vi "新剖面数据上传.vi"(11 "错误输入（无错误）":errorcluster) -> (15 "error out":errorcluster)   [LabVIEW 2016, in "数据传输系统-02.lvlib"]
uses:
  <vilib>/Utility/config.llb/Write Key (String).vi
  <vilib>/Utility/config.llb/Read Key (String).vi
  <vilib>/Utility/config.llb/NI_LVConfig.lvlib
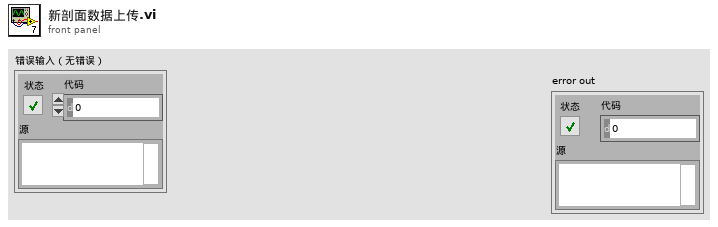
[diagram p1: front panel]
types:
  T1 = cluster{"setini":string, "sysini":string, "hechaini":string, "actualwrite":string, "actualread":string, "datasent":string, "反控命令信息队列":string, "反控与仪器交互":string}
  T2 = typedef "NI_LVConfig.lvlib/Config Data RefNum.ctl" = refnum<k1>
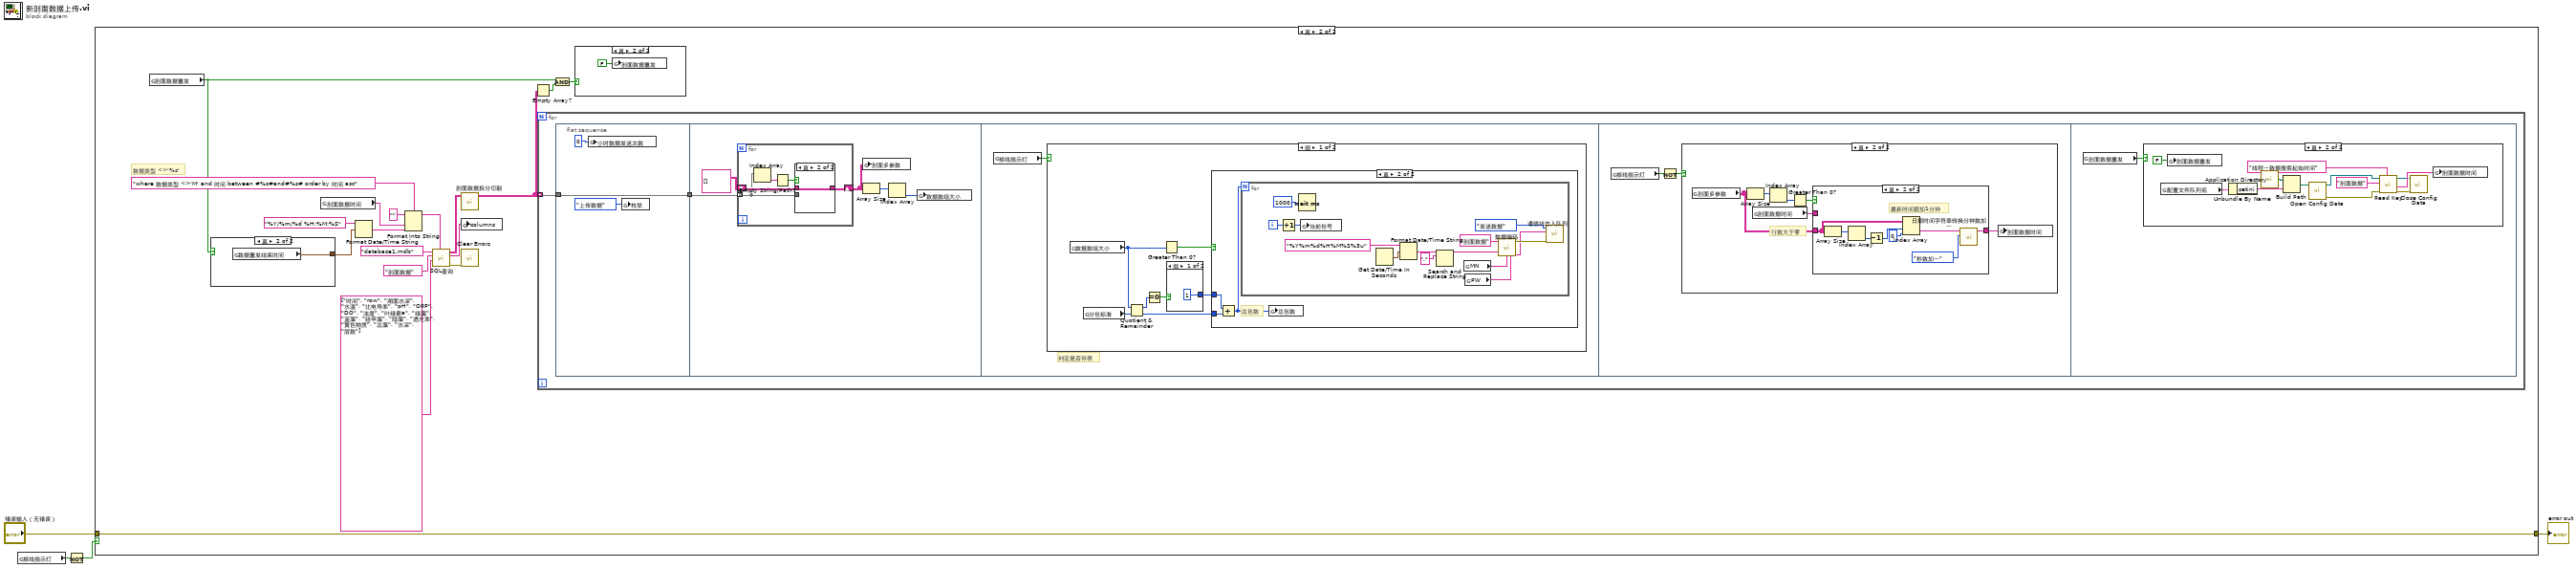
[diagram p0: block diagram]
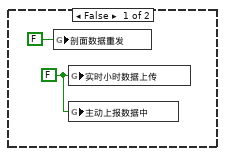
[diagram p2: hidden frame]
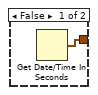
[diagram p4: hidden frame]
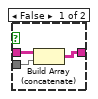
[diagram p5: hidden frame]
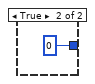
[diagram p6: hidden frame]
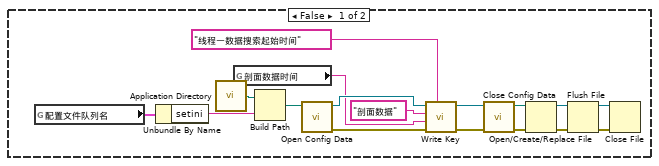
[diagram p11: hidden frame]
diagram:
  n1 = global read "全局 数据发送重叠.vi" "掉线指示灯"() -> (w4:bool)
  n2 = Not(x=w4) -> (.not. x?=w1:bool)
  n3 = case shown="真" w1 {
    tunnel: [_ w24] -> w3
    tunnel: "错误输入（无错误）" -> [_ w24]
    frame False {
      w6 = FALSE ("小时数据上传")
      n4 = global write "断电保存全局.vi" "剖面数据重发"(FALSE ("剖面数据重发")) -> ()
      n5 = global write "全局1.vi" "实时小时数据上传"(w6) -> ()
      n6 = global write "全局 数据发送重叠.vi" "主动上报数据中"(w6) -> ()
    }
    frame True {
      # "数据类型 <>'%s'"
      n7 = global read "断电保存全局.vi" "剖面数据重发"() -> (w7:bool)
      n8 = case shown="真" w7 {
        tunnel: [w26 w27] -> w11
        frame False {
          n9 = Get Date/Time In Seconds() -> (seconds since 1Jan1904=w26:timestamp)
        }
        frame True {
          n10 = global read "断电保存全局.vi" "数据重发结束时间"() -> (w27:timestamp)
        }
      }
      n11 = global read "全局 水样时间.vi" "剖面数据时间"() -> (w17:string)
      n12 = Format Date/Time String(time format string (%c)="%Y/%m/%d %H:%M:%S" ("时间格式字符串(%c)"), seconds (now)=w11) -> (date/time string=w16:string)  [unwired: 1 in]
      n13 = Format Into String(format string="where 数据类型 <>'M' and 时间 between #%s#and#%s# order by 时间 asc" ("condition"), initial string="" ("初始字符串"), w17, w16) -> (resulting string=w15:string)  [unwired: 1 in, 1 out]
      n14 = call "SQL查询.vi"("condition"=w15, "columns"=string[] ["时间", "row", "湖面水深", "水温", "比电导率", "pH", "ORP", "DO", "浊度", "叶绿素a", "绿藻", "蓝藻", "硅甲藻", "隐藻", "透光率", "黄色物质", "总藻", "水深", "层数"], "table输入"="剖面数据", "database"="database1.mdb") -> ("error out"=w13:errorcluster, "columns输出"=w14:string[], "data"=w23:string[][])  [unwired: 4 in, 1 out]
      n15 = call "剖面数据拆分切割.vi"("剖面多参数输入"=w23) -> ("剖面多参数输出"=w10:string[][][])  [unwired: 10 in]
      n16 = global write "全局 所有参数.vi" "columns"(w14) -> ()
      n17 = call <vilib>:"Clear Errors.vi"("error in (no error)"=w13) -> ()  [unwired: 5 in, 2 out]
      n18 = Empty Array?(array=w10) -> (empty?=w9:bool)
      n19 = for {
        tunnel: w10 -> [w29] mode=indexing
        n20 = flat-sequence {
          tunnel: w29 -> [w32]
          tunnel: [w32] -> w28
          tunnel: w28 -> [w35]
          frame #0 {
            n21 = global write "全局 小时数据发送次数.vi" "小时数据发送次数"(0 ("小时数据发送次数")) -> ()
            n22 = global write "全局1.vi" "枚举"(enum16{"返回请求应答", "上传数据", "返回执行结果"}."上传数据" ("枚举")) -> ()
          }
          frame #1 {
            n23 = for {
              tunnel: w35 -> [w40] mode=indexing
              shift-right: [w41] -> w33
              shift-left: string[][] [] ("剖面多参数输入") -> [w42]
              n24 = Index Array(array=w40) -> (element=w39:string)  [unwired: 1 in]
              n25 = Empty String/Path?(string/path=w39) -> (empty?=w38:bool)
              n26 = case shown="真" w38 {
                tunnel: w42 -> [w45 w46]
                tunnel: w40 -> [w44 _]
                tunnel: [w43 w46] -> w41
                frame False {
                  n27 = Build Array (concatenate)(w45, w44) -> (w43:string[][])
                }
                frame True {
                }
              }
            }
            n28 = global write "全局 所有参数.vi" "剖面多参数"(w33) -> ()
            n29 = Array Size(array=w33) -> (size(s)=w36:i32[])
            n30 = Index Array(array=w36) -> (element=w37:i32)  [unwired: 1 in]
            n31 = global write "全局 数据数组大小.vi" "数据数组大小"(w37) -> ()
          }
          frame #2 {
            # "判定是否存表"
            n32 = global read "全局 数据发送重叠.vi" "掉线指示灯"() -> (w47:bool)
            n33 = case shown="假" w47 {
              frame False {
                n34 = global read "全局 数据数组大小.vi" "数据数组大小"() -> (w53:i32)
                n35 = global read "全局 数据数组大小.vi" "分包标准"() -> (w51:i32)
                n36 = Quotient & Remainder(x=w53, y=w51) -> (x-y*floor(x/y)=w50:i32, floor(x/y)=w52:i32)
                n37 = Equal To 0?(x=w50) -> (x = 0?=w49:bool)
                n38 = Greater Than 0?(x=w53) -> (x > 0?=w54:bool)
                n39 = case shown="假" w49 {
                  tunnel: [1 ("x") 0 ("x")] -> w48
                  frame False {
                  }
                  frame True {
                  }
                }
                n40 = case shown="真" w54 {
                  tunnel: w52 -> [_ w59]
                  tunnel: w48 -> [_ w57]
                  frame False {
                  }
                  frame True {
                    # "总包数"
                    n41 = Add(x=w57, y=w59) -> (x+y=w58:i32)
                    n42 = for {
                      N: w58 -> [_]
                      i -> [w63]
                      n43 = Increment(x=w63) -> (x+1=w62:i32)
                      n44 = Wait (ms)(milliseconds to wait=u32 1000 ("等待时间（毫秒）")) -> ()  [unwired: 1 out]
                      n45 = global write "全局 数据数组大小.vi" "当前包号"(w62) -> ()
                      n46 = Get Date/Time In Seconds() -> (seconds since 1Jan1904=w71:timestamp)
                      n47 = Format Date/Time String(time format string (%c)="%Y%m%d%H%M%S%3u" ("时间格式字符串(%c)"), seconds (now)=w71) -> (date/time string=w70:string)  [unwired: 1 in]
                      n48 = Search and Replace String(input string=w70, search string="." ("搜索字符串")) -> (result string=w68:string)  [unwired: 6 in, 3 out]
                      n49 = global read "断电保存全局.vi" "MN"() -> (w67:string)
                      n50 = global read "断电保存全局.vi" "PW"() -> (w66:string)
                      n51 = call "数据编码.vi"("table输入"="剖面数据" ("新元素/子数组"), "QN"=w68, "MN"=w67, "PW"=w66) -> ("错误常量"=w65:errorcluster, "通讯包字符串"=w60:string)  [unwired: 10 in]
                      n52 = call "通信状态入队列.vi"("错误输入（无错误）"=w65, "发送报文"=w60, "枚举"=enum16{"打开连接", "发送数据", "读取数据", "数据处理", "关闭连接"}."发送数据") -> ()  [unwired: 8 in, 1 out]
                    }
                    n53 = global write "全局 数据数组大小.vi" "总包数"(w58) -> ()
                  }
                }
              }
              frame True {
              }
            }
          }
          frame #3 {
            n54 = global read "全局 数据发送重叠.vi" "掉线指示灯"() -> (w74:bool)
            n55 = Not(x=w74) -> (.not. x?=w75:bool)
            n56 = case shown="真" w75 {
              frame False {
              }
              frame True {
                # "行数大于零"
                n57 = global read "全局 所有参数.vi" "剖面多参数"() -> (w80:string[][])
                n58 = Array Size(array=w80) -> (size(s)=w77:i32[])
                n59 = global read "全局 水样时间.vi" "剖面数据时间"() -> (w81:string)
                n60 = Index Array(array=w77) -> (element=w78:i32)  [unwired: 1 in]
                n61 = Greater Than 0?(x=w78) -> (x > 0?=w79:bool)
                n62 = case shown="真" w79 {
                  tunnel: w80 -> [_ w87]
                  tunnel: [w82 w84] -> w76
                  tunnel: w81 -> [w82 _]
                  frame False {
                  }
                  frame True {
                    # "最新时间戳加1分钟"
                    n63 = Array Size(array=w87) -> (size(s)=w89:i32[])
                    n64 = Index Array(array=w89) -> (element=w88:i32)  [unwired: 1 in]
                    n65 = Decrement(x=w88) -> (x-1=w86:i32)
                    n66 = Index Array(array=w87, index (row)=w86, index (col)=0 ("禁用的索引 (列)")) -> (element=w90:string)
                    n67 = call "日期时间字符串转换分钟数加一.vi"("枚举"=enum16{"分钟数加一", "秒数加一", "小时数加一"}."秒数加一", "data[0]"=w90) -> ("日期/时间字符串"=w84:string)  [unwired: 9 in]
                  }
                }
                n68 = global write "全局 水样时间.vi" "剖面数据时间"(w76) -> ()
              }
            }
          }
          frame #4 {
            n69 = global read "断电保存全局.vi" "剖面数据重发"() -> (w91:bool)
            n70 = case shown="真" w91 {
              frame False {
                n71 = global read "断电保存全局.vi" "配置文件队列名"() -> (w93:T1)
                n72 = Unbundle By Name(w93) -> ("setini"=w92:string)
                n73 = call <vilib>:"Application Directory.vi"() -> ("Application Directory"=w102:path)
                n74 = global read "全局 水样时间.vi" "剖面数据时间"() -> (w94:string)
                n75 = Build Path(base path=w102, name or relative path=w92) -> (appended path=w103:path)
                n76 = call <vilib>:"Open Config Data.vi"("configuration file path"=w103) -> ("error out"=w105:errorcluster, "refnum"=w104:T2)  [unwired: 8 in, 1 out]
                n77 = call-poly <vilib>:"Write Key.vi"("section"="线程一数据搜索起始时间", "error in (no error)"=w105, "value"=w94, "key"="剖面数据", "refnum"=w104) -> ("error out"=w107:errorcluster, "refnum out"=w106:T2)  [unwired: 4 in, 1 out]
                n78 = call <vilib>:"Close Config Data.vi"("error in (no error)"=w107, "refnum"=w106) -> ("error out"=w95:errorcluster, "file path"=w96:path)  [unwired: 8 in]
                n79 = Open/Create/Replace File(file path (use dialog)=w96, error in=w95) -> (refnum out=w98:refnum<file>, error out=w97:errorcluster)  [unwired: 4 in, 1 out]
                n80 = Flush File(refnum=w98, error in=w97) -> (refnum out=w99:refnum<file>, error out=w100:errorcluster)
                n81 = Close File(refnum=w99, error in=w100) -> ()  [unwired: 2 out]
              }
              frame True {
                n82 = global read "断电保存全局.vi" "配置文件队列名"() -> (w116:T1)
                n83 = global write "断电保存全局.vi" "剖面数据重发"(FALSE ("剖面数据重发")) -> ()
                n84 = Unbundle By Name(w116) -> ("setini"=w117:string)
                n85 = call <vilib>:"Application Directory.vi"() -> ("Application Directory"=w115:path)
                n86 = Build Path(base path=w115, name or relative path=w117) -> (appended path=w118:path)
                n87 = call <vilib>:"Open Config Data.vi"("configuration file path"=w118) -> ("error out"=w112:errorcluster, "refnum"=w111:T2)  [unwired: 8 in, 1 out]
                n88 = call-poly <vilib>:"Read Key.vi"("section"="线程一数据搜索起始时间", "error in (no error)"=w112, "key"="剖面数据", "refnum"=w111) -> ("error out"=w114:errorcluster, "value"=w120:string, "refnum out"=w113:T2)  [unwired: 4 in, 1 out]
                n89 = call <vilib>:"Close Config Data.vi"("error in (no error)"=w114, "refnum"=w113) -> ()  [unwired: 8 in, 2 out]
                n90 = global write "全局 水样时间.vi" "剖面数据时间"(w120) -> ()
              }
            }
          }
        }
      }
      n91 = And(x=w7, y=w9) -> (x .and. y?=w8:bool)
      n92 = case shown="真" w8 {
        frame False {
        }
        frame True {
          n93 = global write "断电保存全局.vi" "剖面数据重发"(FALSE ("剖面数据重发")) -> ()
        }
      }
    }
  }
  "error out" <- w3
